vi "Encoder to Inch.vi"(5 "Encoder in":i32) -> (6 "Encoder out(in)":dbl)   [LabVIEW 2015, in "Tool Cfg.lvlib"]
uses:
  Tool Cfg.lvlib
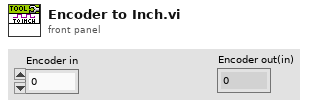
[diagram p1: front panel]
types:
  T1 = typedef "Tool Cfg.lvlib/_Tool Block Cluster_v3--typedef.ctl" = cluster{"Encoder Size":u16, "Encoder Scale":u32, "Encoder Offset":i32, "MaxEncoder":i32, "MinEncoder":i32, "Start Delay":sgl, "Tool Face Ref":sgl}
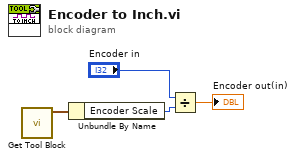
[diagram p0: block diagram]
diagram:
  n1 = call "Get Tool Block.vi"() -> ("Tool Block"=w3:T1)  [unwired: 11 in]
  n2 = Unbundle By Name(w3) -> ("Encoder Scale"=w2:u32)
  n3 = Divide(x="Encoder in", y=w2) -> (x/y=→"Encoder out(in)":dbl)
